vi "Get GPS Waypoints.vi"(11 "File name":string) -> (3 "GPS Waypoints":T1[](array[typedef]) {"Longitude" format="%#_14g"; "Latitude" format="%#_14g"})   [LabVIEW 2009]
uses:
  TypeDefs/Sensor Typedefs/GPS Data.ctl
panel:
  in  "error in":errorcluster
  out "error out":errorcluster
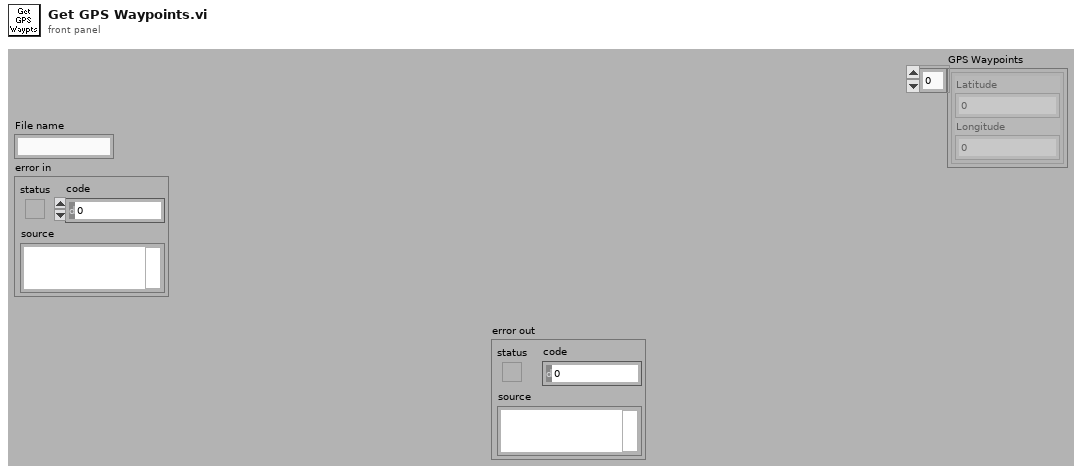
[diagram p1: front panel]
types:
  T1 = typedef "GPS Data.ctl" = cluster{"Latitude":dbl, "Longitude":dbl}
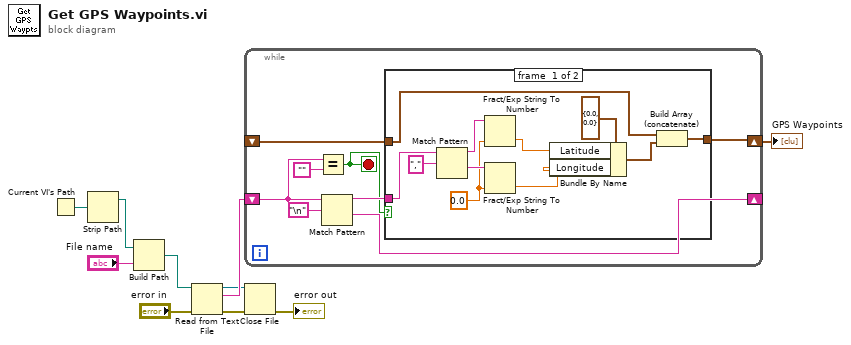
[diagram p0: block diagram]
diagram:
  n1 = Current VI's Path() -> (path=w2:path)
  n2 = Strip Path(path=w2) -> (stripped path=w3:path)  [unwired: 1 out]
  n3 = Build Path(base path=w3, name or relative path="File name") -> (appended path=w5:path)
  n4 = Read from Text File(file (use dialog)=w5, error in="error in") -> (refnum out=w7:refnum<file>, text=w10:string, error out=w8:errorcluster)  [unwired: 3 out]
  n5 = while {
    shift-right: [w14] -> _
    shift-left: w10 -> [w17]
    shift-right: [w11] -> w1
    shift-left: _ -> [w12]
    stop <- w15 stop-if-true
    n6 = Equal?(x=w17, y="") -> (x = y?=w15:bool)
    n7 = Match Pattern(string=w17, regular expression="\n") -> (before substring=w18:string, after substring=w14:string)  [unwired: 1 in, 2 out]
    n8 = case shown="False" w15 {
      tunnel: w18 -> [w28 _]
      tunnel: w12 -> [w19 w30]
      tunnel: [w20 w30] -> w11
      frame #0 {
        w25 = 0.0
        n9 = Match Pattern(string=w28, regular expression=",") -> (before substring=w27:string, after substring=w26:string)  [unwired: 1 in, 2 out]
        n10 = Fract/Exp String To Number(string=w27, default (0 dbl)=w25) -> (number=w24:dbl)  [unwired: 3 out]
        n11 = Fract/Exp String To Number(string=w26, default (0 dbl)=w25) -> (number=w23:dbl)  [unwired: 3 out]
        n12 = Bundle By Name(cluster=T1 {"Latitude"=0.0, "Longitude"=0.0} ("GPS Point"), "Latitude"=w24, "Longitude"=w23) -> (w22:T1)
        n13 = Build Array (concatenate)(w19, w22) -> (w20:T1[])
      }
      frame #1 {
      }
    }
  }
  "GPS Waypoints" <- w1
  n14 = Close File(refnum=w7, error in=w8) -> (error out=→"error out":errorcluster)  [unwired: 1 out]
